vi "Write to File.vi"(8 "error in (no error)":errorcluster, 10 "INI Ref":T1, 11 "Disabled Assertion in":refnum<class "Disabled Assertion.lvclass">) -> (0 "error out":errorcluster, 2 "INI Ref out":T1, 3 "Disabled Assertion out":refnum<class "Disabled Assertion.lvclass">)   [LabVIEW 2020, in "MacroAssert.lvlib" / "Disabled Assertion.lvclass"]
uses:
  Disabled Assertion.lvclass
  Disabled Assertion.lvclass/Disabled Assertion.ctl
  Control Assertion/Control Assertion.lvclass
  MacroAssert.lvlib
  <vilib>/Utility/config.llb/NI_LVConfig.lvlib
  <vilib>/Utility/config.llb/Write Key (String).vi
  <vilib>/Utility/config.llb/Config Data RefNum.ctl
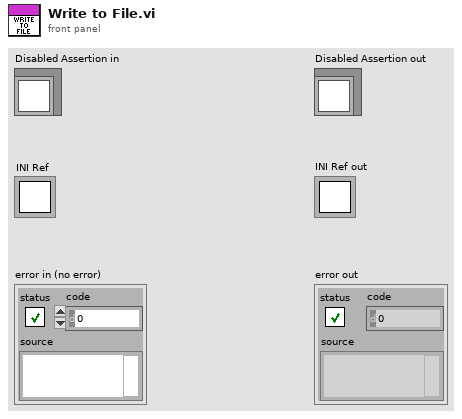
[diagram p1: front panel]
types:
  T1 = typedef "NI_LVConfig.lvlib/Config Data RefNum.ctl" = refnum<k1>
  T2 = enum8{"Enabled", "Disabled", "Disabled and Grayed Out"}
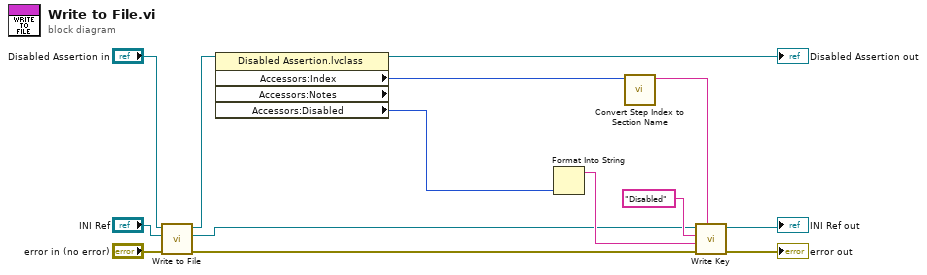
[diagram p0: block diagram]
diagram:
  n1 = call-parent "Write to File.vi"("error in (no error)"="error in (no error)", "INI Ref"="INI Ref", "Control Assertion in"="Disabled Assertion in") -> ("error out"=w6:errorcluster, "INI Ref out"=w2:T1, "Control Assertion out"=w5:refnum<class "Disabled Assertion.lvclass">)  [unwired: 6 in]
  n2 = property class="Disabled Assertion.lvclass" props=["Accessors:Index", "Accessors:Notes", "Accessors:Disabled"](reference=w5) -> (reference out=→"Disabled Assertion out":refnum<class "Disabled Assertion.lvclass">, "Accessors:Index"=w10:i32, "Accessors:Disabled"=w8:T2)  [unwired: 1 in, 2 out]
  n3 = Format Into String(w8) -> (resulting string=w7:string)  [unwired: 3 in, 1 out]
  n4 = call "Convert Step Index to Section Name.vi"("Step Index"=w10) -> ("Section Name"=w9:string)  [unwired: 10 in]
  n5 = call-poly <vilib>:"Write Key.vi"("section"=w9, "error in (no error)"=w6, "value"=w7, "key"="Disabled", "refnum"=w2) -> ("error out"=→"error out":errorcluster, "refnum out"=→"INI Ref out":T1)  [unwired: 4 in, 1 out]
